vi "PWM Encoder Reading for NXT motors.vi"() -> ()   [LabVIEW 2013]
uses:
  <vilib>/eio/EIONode/EIONode.xnode
  <vilib>/rvi/eio/common/nirviEmuTemplateMethod_errors.vi
panel:
  in  "Tab Control":enum32{"Page 1", "Page 2"}(tab)
  in  "Control":T1={"Pulse Lenght DIO3"=10000, "Pulse Period 3"=20000, "Dephasing 3"=0, "Pulse Lenght DIO0"=10000, "Pulse Period 0"=20000, "Dephasing 0"=0}
  in  "Update":bool
  out "Cluster":T1
  out "Velocity (Counts/Interval)":i64
  out "Acceleration (Counts/Interval)":i64
  in  "Velocity Interval (uSec)":u32
  out "Position (Counts)":u64
  in  "Position Reset":bool
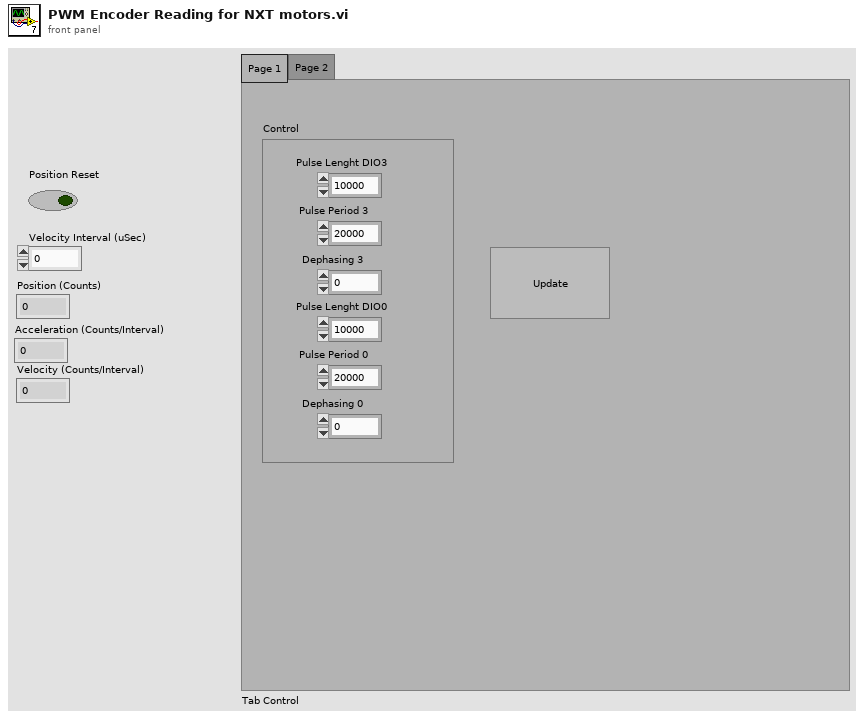
[diagram p1: front panel]
types:
  T1 = cluster{"Pulse Lenght DIO3":i16, "Pulse Period 3":i16, "Dephasing 3":i16, "Pulse Lenght DIO0":i16, "Pulse Period 0":i16, "Dephasing 0":i16}
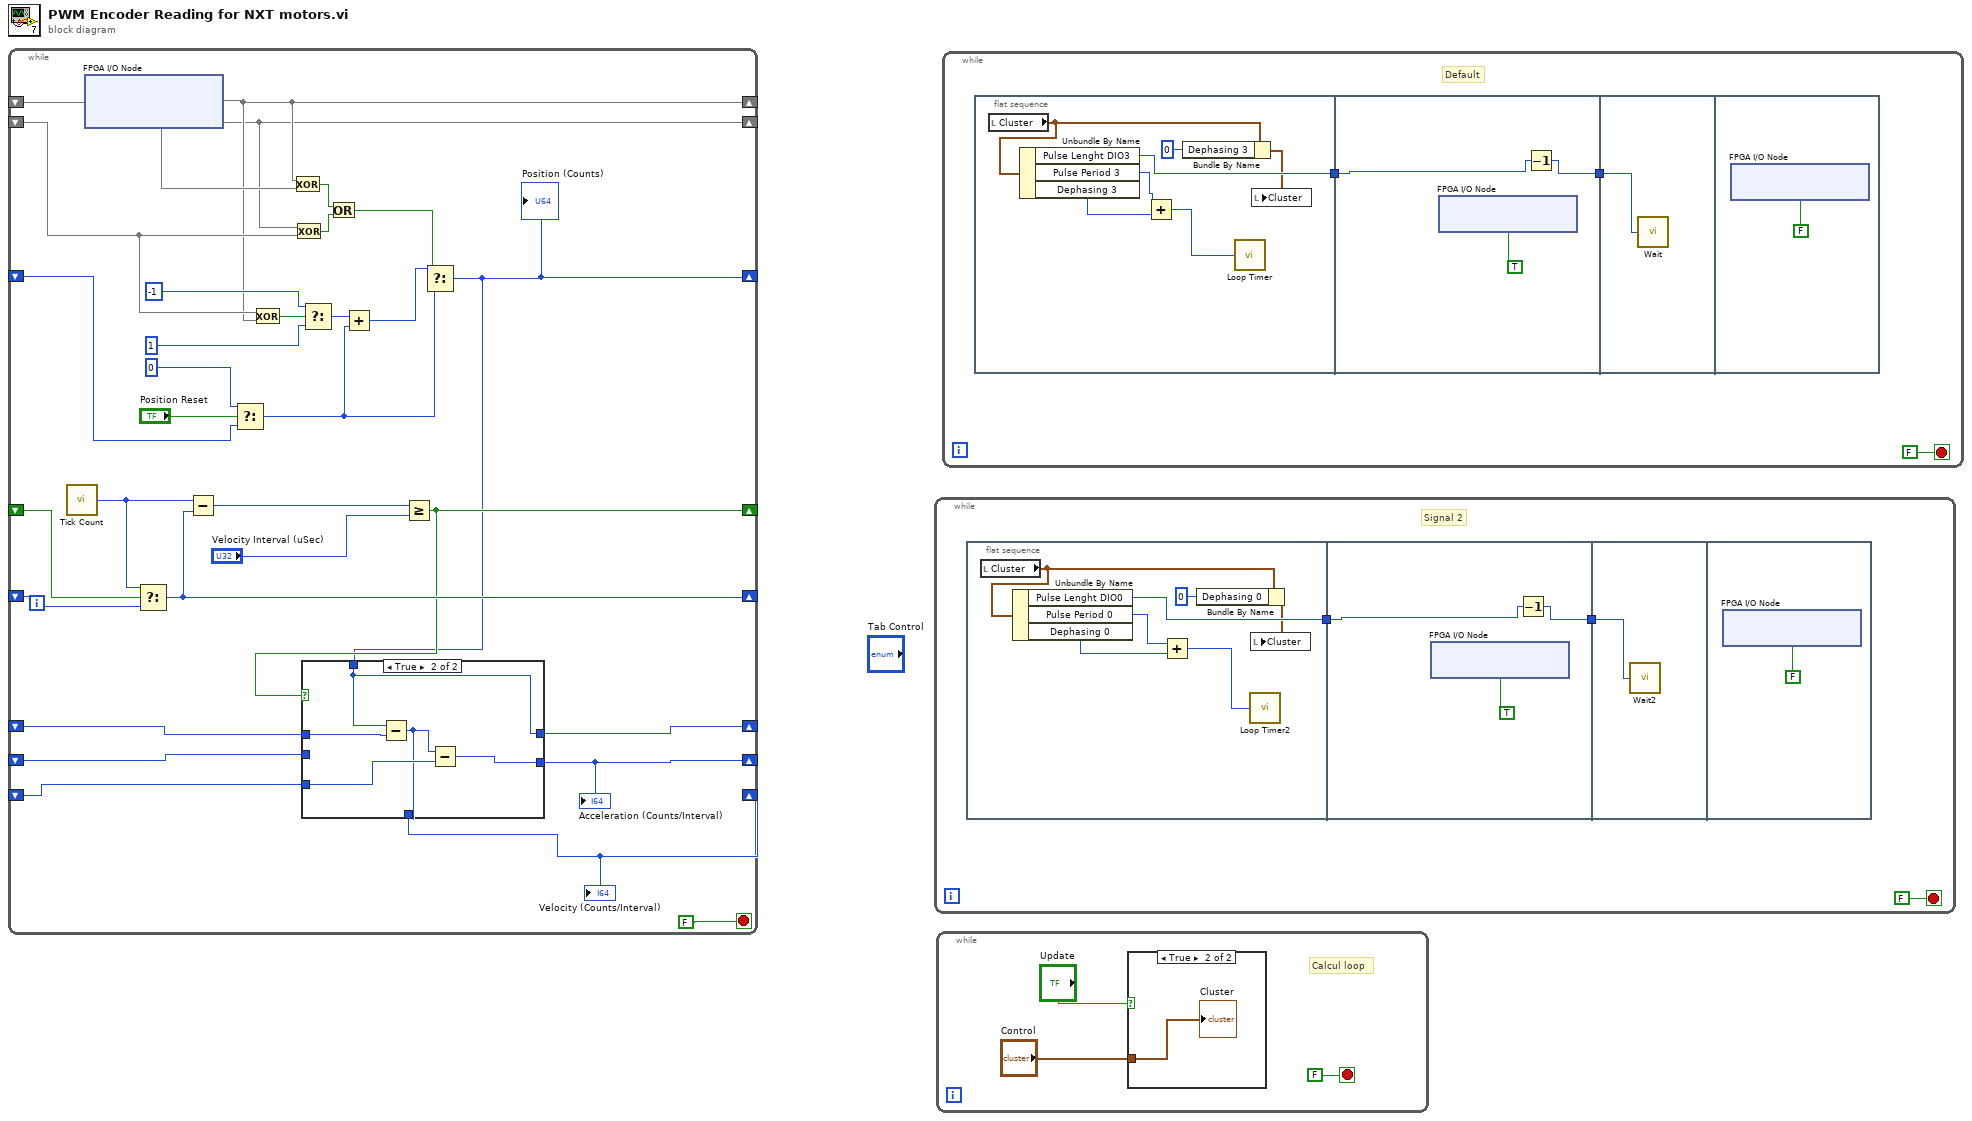
[diagram p0: block diagram]
diagram:
  n1 = while {
    shift-right: [w4] -> _
    shift-left: _ -> [w31]
    shift-right: [w3] -> _
    shift-left: _ -> [w5]
    shift-right: [w12] -> _
    shift-left: _ -> [w24]
    shift-right: [w14] -> _
    shift-left: _ -> [w17]
    shift-right: [w15] -> _
    shift-left: _ -> [w16]
    shift-right: [w11] -> _
    shift-left: _ -> [w13]
    shift-right: [w10] -> _
    shift-left: _ -> [w7]
    shift-right: [w8] -> _
    shift-left: _ -> [w9]
    stop <- FALSE stop-if-true
    n2 = call "Tick Count"() -> ("Tick Count(Ticks)"=w19:u32)
    n3 = xnode "FPGA I/O Node"() -> ("ConnectorA/DIO6"=w4, "ConnectorA/DIO7"=w3)  [unwired: 2 in, 2 out]
    n4 = Select(t=w19, s=w17, f=w16) -> (s? t:f=w15:u32)
    n5 = Subtract(x=w19, y=w15) -> (x-y=w20:u32)
    n6 = Select(t=i16 0, s="Position Reset", f=w24) -> (s? t:f=w21:i16)
    n7 = Exclusive Or(1:w4, 2:w5) -> (0:w2:bool)
    n8 = Exclusive Or(1:w31, 2:w4) -> (0:w30:bool)
    n9 = Exclusive Or(1:w5, 2:w3) -> (0:w29:bool)
    n10 = Select(t=i16 -1, s=w2, f=i16 1) -> (s? t:f=w23:i16)
    n11 = Or(x=w30, y=w29) -> (x .or. y?=w28:bool)
    n12 = Add(x=w23, y=w21) -> (x+y=w22:i16)
    n13 = Greater Or Equal?(x=w20, y="Velocity Interval (uSec)") -> (x >= y?=w14:bool)
    n14 = Select(t=w22, s=w28, f=w21) -> (s? t:f=w12:i16)
    "Position (Counts)" <- w12
    n15 = case shown="True" w14 {
      tunnel: w13 -> [w34 w39]
      tunnel: w12 -> [_ w38]
      tunnel: [w34 w38] -> w11
      tunnel: [w33 w37] -> w10
      tunnel: w9 -> [w32 w36]
      tunnel: [w32 w35] -> w8
      tunnel: w7 -> [w33 _]
      frame False {
      }
      frame True {
        n16 = Subtract(x=w38, y=w39) -> (x-y=w35:i16)
        n17 = Subtract(x=w35, y=w36) -> (x-y=w37:i16)
      }
    }
    "Acceleration (Counts/Interval)" <- w10
    "Velocity (Counts/Interval)" <- w8
  }
  n18 = while {
    stop <- FALSE stop-if-true
    # "Signal 2"
    n19 = flat-sequence {
      tunnel: [w49] -> w41
      tunnel: w41 -> [w50]
      tunnel: [w51] -> w40
      tunnel: w40 -> [w53]
      frame #0 {
        n20 = local read "Cluster"() -> (w48:T1)
        n21 = Unbundle By Name(w48) -> ("Pulse Lenght DIO0"=w49:i16, "Pulse Period 0"=w45:i16, "Dephasing 0"=w44:i16)
        n22 = Add(x=w45, y=w44) -> (x+y=w43:i16)
        n23 = Bundle By Name(cluster=w48, "Dephasing 0"=i16 0 ("Dephasing 3")) -> (w46:T1)
        n24 = call "Loop Timer2"("Count(Ticks)"=w43) -> ()  [unwired: 1 out]
        n25 = local write "Cluster"(w46) -> ()
      }
      frame #1 {
        n26 = xnode "FPGA I/O Node"("ConnectorC/DIO0"=TRUE ("ConnectorC/DIO7")) -> ()  [unwired: 1 in, 1 out]
        n27 = Decrement(x=w50) -> (x-1=w51:i16)
      }
      frame #2 {
        n28 = call "Wait2"("Count(Ticks)"=w53) -> ()  [unwired: 1 out]
      }
      frame #3 {
        n29 = xnode "FPGA I/O Node"("ConnectorC/DIO0"=FALSE ("ConnectorC/DIO7")) -> ()  [unwired: 1 in, 1 out]
      }
    }
  }
  n30 = while {
    stop <- FALSE stop-if-true
    # "Calcul loop"
    n31 = case shown="True" "Update" {
      tunnel: "Control" -> [_ w58]
      frame False {
      }
      frame True {
        "Cluster" <- w58
      }
    }
  }
  n32 = while {
    stop <- FALSE stop-if-true
    # "Default"
    n33 = flat-sequence {
      tunnel: [w68] -> w60
      tunnel: w60 -> [w69]
      tunnel: [w70] -> w59
      tunnel: w59 -> [w72]
      frame #0 {
        n34 = local read "Cluster"() -> (w62:T1)
        n35 = Unbundle By Name(w62) -> ("Pulse Lenght DIO3"=w68:i16, "Pulse Period 3"=w66:i16, "Dephasing 3"=w67:i16)
        n36 = Add(x=w66, y=w67) -> (x+y=w65:i16)
        n37 = Bundle By Name(cluster=w62, "Dephasing 3"=i16 0) -> (w63:T1)
        n38 = call "Loop Timer"("Count(Ticks)"=w65) -> ()  [unwired: 1 out]
        n39 = local write "Cluster"(w63) -> ()
      }
      frame #1 {
        n40 = xnode "FPGA I/O Node"("ConnectorC/DIO3"=TRUE ("ConnectorC/DIO7")) -> ()  [unwired: 1 in, 1 out]
        n41 = Decrement(x=w69) -> (x-1=w70:i16)
      }
      frame #2 {
        n42 = call "Wait"("Count(Ticks)"=w72) -> ()  [unwired: 1 out]
      }
      frame #3 {
        n43 = xnode "FPGA I/O Node"("ConnectorC/DIO3"=FALSE ("ConnectorC/DIO7")) -> ()  [unwired: 1 in, 1 out]
      }
    }
  }
